vi "Team Stats.vi"(8 "error in (no error)":errorcluster, 11 "Game in":refnum<class "Game.lvclass">) -> (0 "error out":errorcluster, 1 "Won?":bool, 2 "Team Stats":T1[](array[typedef]), 3 "Game out":refnum<class "Game.lvclass">)   [LabVIEW 2020, in "SquareBattle.lvlib" / "Game.lvclass"]
uses:
  Game.lvclass
  SB App/Team Status Data.ctl
  Team Stats.ctl
  Team State.ctl
  Game.lvclass/Game.ctl
  SquareBattle.lvlib
  SB App/SB App.lvlib
  Team/Team.lvclass
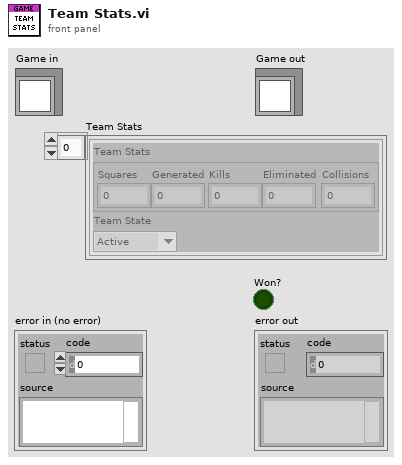
[diagram p1: front panel]
types:
  T1 = typedef "SB App.lvlib/Team Status Data.ctl" = cluster{"Team Stats":T2, "Team State":T3}
  T2 = typedef "SquareBattle.lvlib/Team Stats.ctl" = cluster{"Squares":i32, "Generated":i32, "Kills":i32, "Eliminated":i32, "Collisions":i32}
  T3 = typedef "SquareBattle.lvlib/Team State.ctl" = enum16{"Active", "Defeated", "Won"}
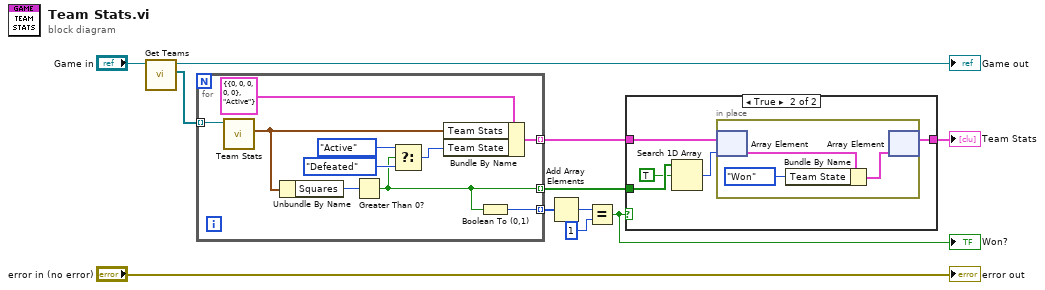
[diagram p0: block diagram]
diagram:
  n1 = call "Get Teams.vi"("Game in"="Game in") -> ("Teams"=w10:refnum<class "Team.lvclass">[], "Game out"=→"Game out":refnum<class "Game.lvclass">)  [unwired: 8 in, 1 out]
  n2 = for {
    tunnel: w10 -> [w21] mode=indexing
    tunnel: [w19] -> w6 mode=indexing
    tunnel: [w13] -> w4 mode=indexing
    tunnel: [w12] -> w9 mode=indexing
    n3 = call "Team Stats.vi"("Team"=w21) -> ("Team Stats"=w18:T2)  [unwired: 10 in]
    n4 = Unbundle By Name(w18) -> ("Squares"=w17:i32)
    n5 = Greater Than 0?(x=w17) -> (x > 0?=w13:bool)
    n6 = Select(t=Team_State."Active" ("Team State"), s=w13, f=Team_State."Defeated" ("Team State")) -> (s? t:f=w14:T3)
    n7 = Bundle By Name(cluster=T1 {"Team Stats"={"Squares"=0, "Generated"=0, "Kills"=0, "Eliminated"=0, "Collisions"=0}, "Team State"=enum."Active"} ("Team Status Data"), "Team Stats"=w18, "Team State"=w14) -> (w19:T1)
    n8 = Boolean To (0,1)(Boolean=w13) -> (0, 1=w12:i16)
  }
  n9 = Add Array Elements(numeric array=w9) -> (sum=w8:i16)
  n10 = Equal?(x=w8, y=i16 1) -> (x = y?=w5:bool)
  "Won?" <- w5
  n11 = case shown="True" w5 {
    tunnel: w6 -> [w22 w25]
    tunnel: w4 -> [_ w27]
    tunnel: [w22 w23] -> w1
    frame False {
    }
    frame True {
      n12 = Search 1D Array(1D array=w27, element=TRUE) -> (index of element=w24:i32)  [unwired: 1 in]
      n13 = in-place {
        n14 = in-place-array #1(w25, w24) -> (w30:T1)
        n15 = Bundle By Name(cluster=w30, "Team State"=Team_State."Won") -> (w28:T1)
        n16 = in-place-array #1(w28) -> (w23:T1[])  [unwired: 1 out]
      }
    }
  }
  "Team Stats" <- w1
  "error out" <- "error in (no error)"
